vi "Append to Data (Dictionary).vi"(8 "error in (no error)":errorcluster, 10 "key-value":cluster{"key":string, "value":variant}, 11 "LVtoITX in":refnum<class "LVtoITX.lvclass">) -> (0 "error out":errorcluster, 3 "LVtoITX out":refnum<class "LVtoITX.lvclass">)   [LabVIEW 2016, in "LVtoITX.lvclass"]
uses:
  LVtoITX.lvclass
  LVtoITX.lvclass/LVtoITX.ctl
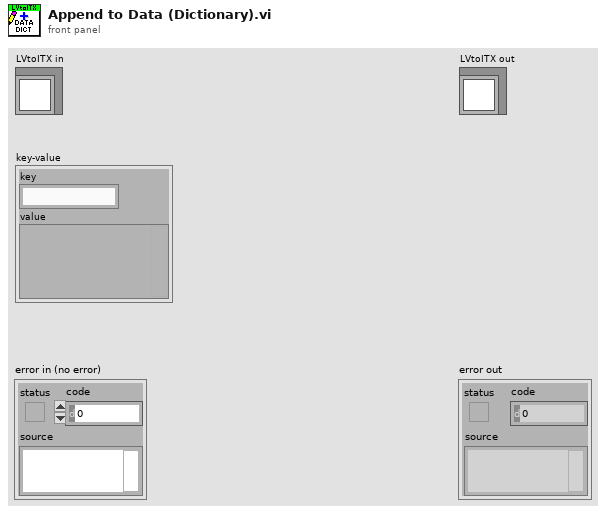
[diagram p1: front panel]
types:
  T1 = typedef "LVtoITX.lvclass/Dictionary--cluster.ctl" = cluster{"key":string, "value":variant}
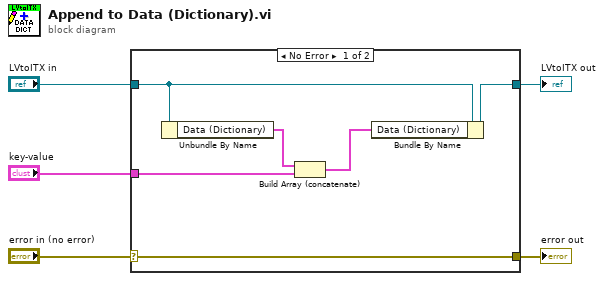
[diagram p0: block diagram]
diagram:
  n1 = case shown="No Error" "error in (no error)" {
    selector: "error in (no error)" -> [w11 w12]
    tunnel: [w11 w12] -> w4
    tunnel: [w10 w13] -> w2
    tunnel: "LVtoITX in" -> [w9 w13]
    tunnel: "key-value" -> [w7 _]
    frame No Error {
      n2 = Unbundle By Name(w9) -> ("Data (Dictionary)"=w8:T1[])
      n3 = Build Array (concatenate)(w8, w7) -> (w6:T1[])
      n4 = Bundle By Name(cluster=w9, "Data (Dictionary)"=w6) -> (w10:refnum<class "LVtoITX.lvclass">)
    }
    frame Error {
    }
  }
  "error out" <- w4
  "LVtoITX out" <- w2
